vi "On Change Configuation Selction.vi"(8 "error in (no error)":errorcluster, 10 "Selection":i32, 11 "App in":refnum<class "App.lvclass">) -> (0 "error out":errorcluster, 3 "App out":refnum<class "App.lvclass">)   [LabVIEW 2020, in "AR Example.lvlib" / "App.lvclass"]
uses:
  App.lvclass
  App.lvclass/App.ctl
  UI/UI.lvclass
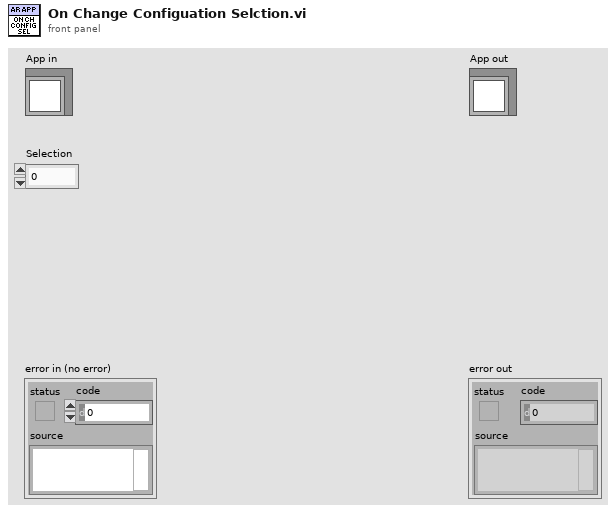
[diagram p1: front panel]
types:
  T1 = typedef "AR Example.lvlib/App.lvclass/JSON Configuration Data.ctl" = cluster{"Version":u32, "Camera Name":string, "Camera Parameters":T2, "Reprojection Error":dbl, "Timestamp":string}
  T2 = typedef "g_ar_toolkit.ar.lvlib/Camera Parameters.ctl" = cluster{"Matrix":T3, "Distortion":T4, "Size":T5}
  T3 = typedef "g_ar_toolkit.ar.lvlib/Camera Matrix.ctl" = cluster{"m 0,0":dbl, "m 0,1":dbl, "m 0,2":dbl, "m 1,0":dbl, "m 1,1":dbl, "m 1,2":dbl, "m 2,0":dbl, "m 2,1":dbl, "m 2,2":dbl}
  T4 = typedef "g_ar_toolkit.ar.lvlib/Camera Distortion Coefficients.ctl" = cluster{"k1":dbl, "k2":dbl, "p1":dbl, "p2":dbl, "k3":dbl, "k4":dbl, "k5":dbl, "k6":dbl, "s1":dbl, "s2":dbl, "s3":dbl, "s4":dbl, "tau x":dbl, "tau y":dbl}
  T5 = typedef "g_ar_toolkit.common.lvlib/Image Size (Integer).ctl" = cluster{"Width":u16, "Height":u16}
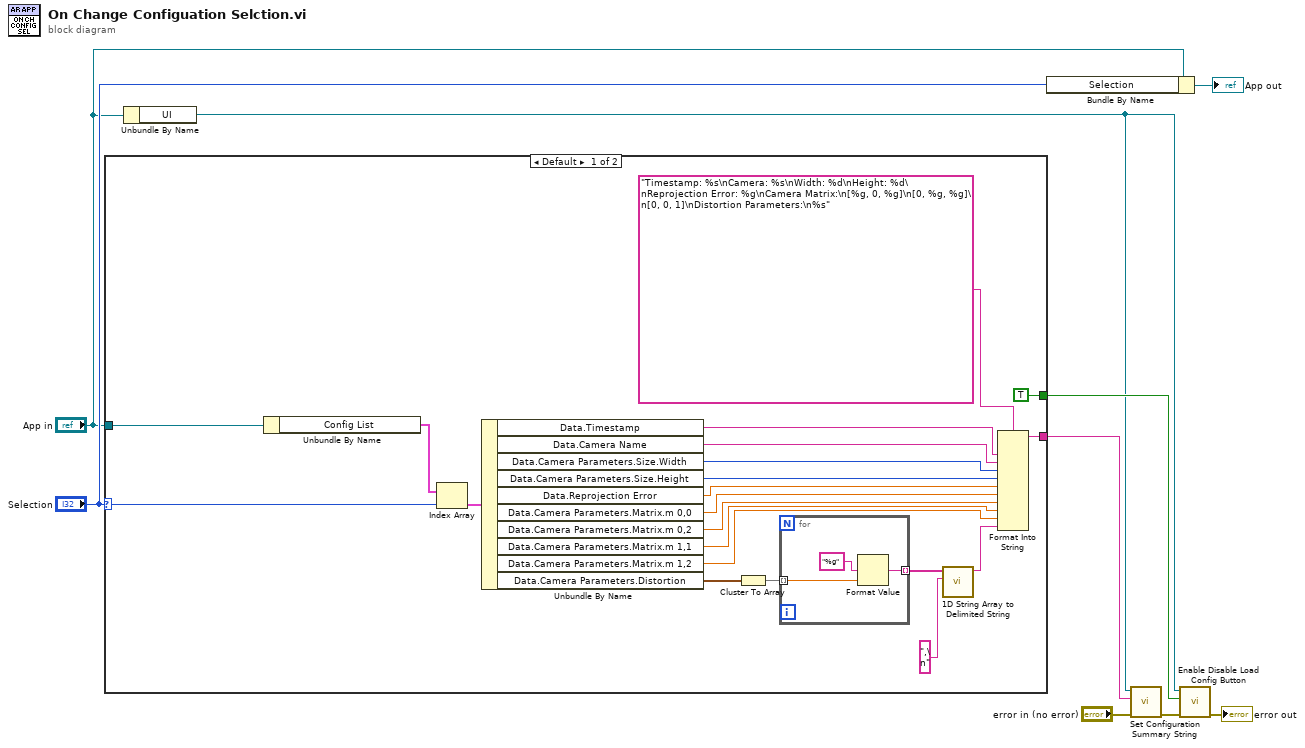
[diagram p0: block diagram]
diagram:
  n1 = case shown="Default" "Selection" {
    selector: "Selection" -> [w25 _]
    tunnel: "App in" -> [w30 _]
    tunnel: [w24 _] -> w6
    tunnel: [TRUE _] -> w5
    frame Default {
      n2 = Unbundle By Name(w30) -> ("Config List"=w29:cluster{"Data":T1, "Source":path}[])
      n3 = Index Array(array=w29, index=w25) -> (element=w26:cluster{"Data":T1, "Source":path})
      n4 = Unbundle By Name(w26) -> ("Data.Timestamp"=w15:string, "Data.Camera Name"=w22:string, "Data.Camera Parameters.Size.Width"=w21:u16, "Data.Camera Parameters.Size.Height"=w28:u16, "Data.Reprojection Error"=w20:dbl, "Data.Camera Parameters.Matrix.m 0,0"=w19:dbl, "Data.Camera Parameters.Matrix.m 0,2"=w18:dbl, "Data.Camera Parameters.Matrix.m 1,1"=w17:dbl, "Data.Camera Parameters.Matrix.m 1,2"=w16:dbl, "Data.Camera Parameters.Distortion"=w14:T4)
      n5 = Cluster To Array(cluster=w14) -> (array=w13:dbl[])
      n6 = for {
        tunnel: w13 -> [w33] mode=indexing
        tunnel: [w31] -> w12 mode=indexing
        n7 = Format Value(format string="%g", value (0)=w33) -> (output string=w31:string)  [unwired: 1 in]
      }
      n8 = call <vilib>:"1D String Array to Delimited String.vi"("delimiter"=",\n", "string array"=w12) -> ("delimited string"=w11:string)  [unwired: 9 in]
      n9 = Format Into String(format string="Timestamp: %s\nCamera: %s\nWidth: %d\nHeight: %d\nReprojection Error: %g\nCamera Matrix:\n[%g, 0, %g]\n[0, %g, %g]\n[0, 0, 1]\nDistortion Parameters:\n%s", w15, w22, w21, w28, w20, w19, w18, w17, w16, w11) -> (resulting string=w24:string)  [unwired: 2 in, 1 out]
    }
    frame -1 {
    }
  }
  n10 = Unbundle By Name("App in") -> ("UI"=w4:refnum<class "UI.lvclass">)
  n11 = Bundle By Name(cluster="App in", "Selection"="Selection") -> (→"App out":refnum<class "App.lvclass">)
  n12 = call-dynamic "Set Configuration Summary String.vi"("error in (no error)"="error in (no error)", "Value"=w6, "UI in"=w4) -> ("error out"=w1:errorcluster)  [unwired: 8 in]
  n13 = call-dynamic "Enable Disable Load Config Button.vi"("error in (no error)"=w1, "Enable?"=w5, "UI in"=w4) -> ("error out"=→"error out":errorcluster)  [unwired: 8 in]
